vi "Resolve Permissions.vi"(8 "error in (no error)":errorcluster, 11 "Authentication Service in":refnum<class "Authentication Service.lvclass">) -> (0 "error out":errorcluster, 3 "Permissions":T1[](array[typedef]))   [LabVIEW 2026, in "Authentication Service.lvclass"]
uses:
  Authentication Service.lvclass
  Authentication Service.lvclass/Authentication Service.ctl
  Domain/Session/Session.lvclass
  Typedefs/enums/Permission Enum.ctl
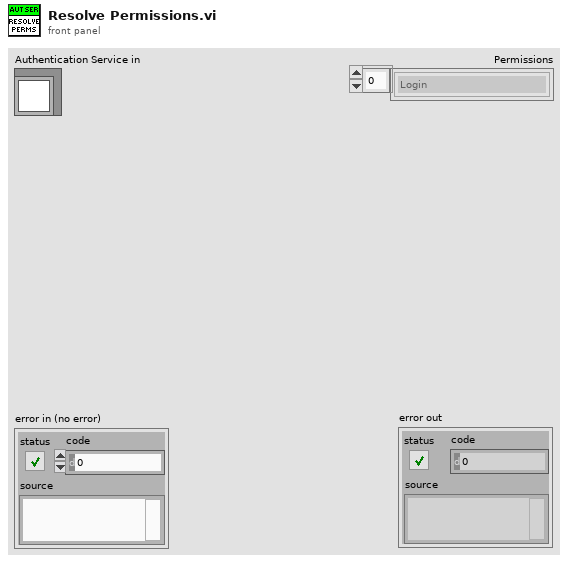
[diagram p1: front panel]
types:
  T1 = typedef "Permission Enum.ctl" = enum16{"Login", "RunReleasedTests", "RunEngineeringTests", "InstallPackages", "UninstallPackages", "EditLocalSettings", "ViewAuditLogs", "ManageUsers", "OverrideWarnings", "ChangeSecurityPolicy"}
  T2 = typedef "Role Enum.ctl" = enum16{"Operator", "Engineer", "Admin"}
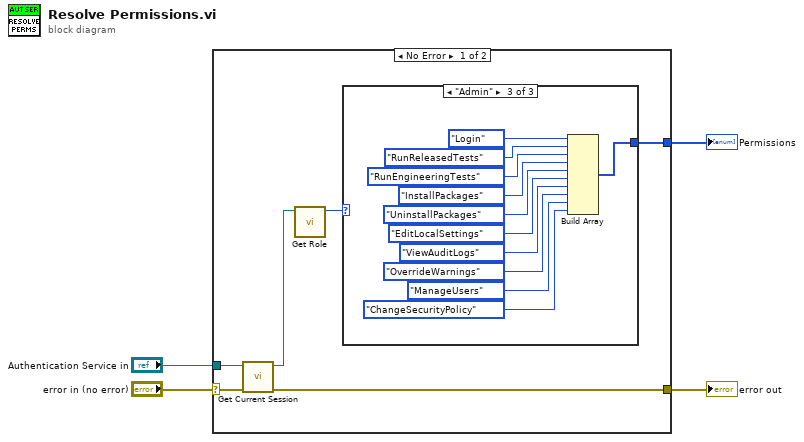
[diagram p0: block diagram]
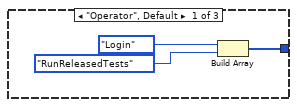
[diagram p2: hidden frame]
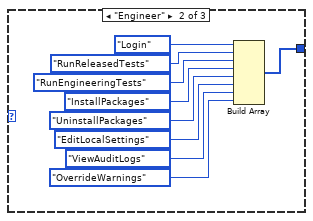
[diagram p3: hidden frame]
diagram:
  n1 = case shown="No Error" "error in (no error)" {
    selector: "error in (no error)" -> [w9 w34]
    tunnel: "Authentication Service in" -> [w10 _]
    tunnel: [w6 _] -> w2
    tunnel: [w5 w34] -> w1
    frame No Error {
      n2 = call "Get Current Session.vi"("error in (no error)"=w9, "Authentication Service"=w10) -> ("error out"=w5:errorcluster, "Current Session"=w8:refnum<class "Session.lvclass">)  [unwired: 8 in]
      n3 = call "Get Role.vi"("Session Data"=w8) -> ("Role"=w7:T2)  [unwired: 10 in]
      n4 = case shown="\"Admin\"" w7 {
        tunnel: [w11 w14 w25] -> w6
        frame "Operator", Default {
          n5 = Build Array(Permission_Enum."Login" ("Permission"), Permission_Enum."RunReleasedTests" ("Permission")) -> (w11:T1[])
        }
        frame "Engineer" {
          n6 = Build Array(Permission_Enum."Login" ("Permission"), Permission_Enum."RunReleasedTests" ("Permission"), Permission_Enum."RunEngineeringTests" ("Permission"), Permission_Enum."InstallPackages" ("Permission"), Permission_Enum."UninstallPackages" ("Permission"), Permission_Enum."EditLocalSettings" ("Permission"), Permission_Enum."ViewAuditLogs" ("Permission"), Permission_Enum."OverrideWarnings" ("Permission")) -> (w14:T1[])
        }
        frame "Admin" {
          n7 = Build Array(Permission_Enum."Login" ("Permission"), Permission_Enum."RunReleasedTests" ("Permission"), Permission_Enum."RunEngineeringTests" ("Permission"), Permission_Enum."InstallPackages" ("Permission"), Permission_Enum."UninstallPackages" ("Permission"), Permission_Enum."EditLocalSettings" ("Permission"), Permission_Enum."ViewAuditLogs" ("Permission"), Permission_Enum."OverrideWarnings" ("Permission"), Permission_Enum."ManageUsers" ("Permission"), Permission_Enum."ChangeSecurityPolicy" ("Permission")) -> (w25:T1[])
        }
      }
    }
    frame Error {
    }
  }
  "error out" <- w1
  "Permissions" <- w2
